vi "SettingsPanel.vi"(8 "error in":errorcluster, 11 "Settings In":T2={"Harware Configuration"={"Camera"="cam1", "Frames Per Second"=15, "Simulate Recording"=FALSE, "Simulated Recording Sample"=path "", "Timestamp Method"=enum."Camera Timestamp"}, "Base Recording Path"=path "", "Type Of Recording"="", "Recording Codec"="", "TrackingSettings"={"Max Radius"=10, "Threshold"=160.0, "ROI"={"Left"=0, "Top"=0, "Right"=0, "Bottom"=0, "Rotation"=0.0}}, "Calibration"={"Pixel Width (X)"=1.0, "Pixel Height (Y)"=1.0}, "Broadcast Length"=0} {"Broadcast Length" min=0; "TrackingSettings"."ROI"."Rotation" format="%.2f"; "TrackingSettings"."ROI"."Left" scale=0.0..1024.0; "TrackingSettings"."ROI"."Right" scale=0.0..1024.0; "TrackingSettings"."Threshold" scale=0.0..255.0}) -> (0 "error out":errorcluster, 2 "Canceled?":bool, 3 "Settings Out":T2={"Harware Configuration"={"Camera"="cam1", "Frames Per Second"=15, "Simulate Recording"=FALSE, "Simulated Recording Sample"=path "", "Timestamp Method"=enum."Camera Timestamp"}, "Base Recording Path"=path "", "Type Of Recording"="", "Recording Codec"="", "TrackingSettings"={"Max Radius"=0, "Threshold"=160.0, "ROI"={"Left"=0, "Top"=0, "Right"=0, "Bottom"=0, "Rotation"=0.0}}, "Calibration"={"Pixel Width (X)"=1.0, "Pixel Height (Y)"=1.0}, "Broadcast Length"=0} {"Broadcast Length" min=0; "TrackingSettings"."ROI"."Rotation" format="%.2f"; "TrackingSettings"."ROI"."Left" scale=0.0..1024.0; "TrackingSettings"."ROI"."Right" scale=0.0..1024.0; "TrackingSettings"."Threshold" scale=0.0..255.0})   [LabVIEW 2017, in "ImageAcquisitionLibrary.lvlib"]
uses:
  ImageAcquisitionLibrary.lvlib
  <vilib>/userdefined/High Color/IMAQdx.ctl
  Settings.ctl
  Tracking/TrackingSettings.ctl
  Calibration.ctl
panel:
  in  "Calibration":T1={"Pixel Width (X)"=1.0, "Pixel Height (Y)"=1.0} {"Pixel Width (X)" format="%.0p"; "Pixel Height (Y)" format="%.0p"}
  in  "Tracking Settings":bool
  in  "Type Of Recording":string(combo)="Snapshot"
  in  "fps":dbl=15.0
  in  "Camera":T3
  in  "Simulate":bool
  in  "Simulated Acquisition Sample":path=path "D:/Dropbox/Colloids/2015-06-15/ImageAcquisitionProgram/SimulationInput/SampleImage.jpg"
  in  "Recording Path":path=path "C:/Users/aortiza/Desktop"
  in  "Codex":string(combo)="Y800 Uncompressed Grey Scale (NI Vision)"
  in  "Cancel Button":bool
  in  "OK Button":bool
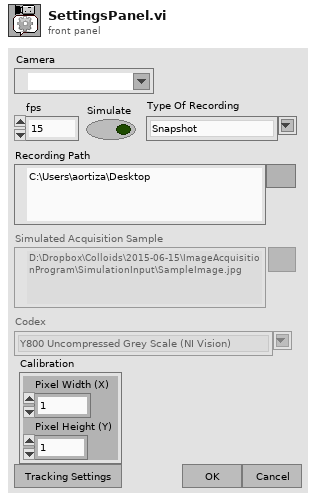
[diagram p1: front panel]
types:
  T1 = typedef "ImageAcquisitionLibrary.lvlib/Calibration.ctl" = cluster{"Pixel Width (X)":dbl, "Pixel Height (Y)":dbl}
  T2 = typedef "ImageAcquisitionLibrary.lvlib/Settings.ctl" = cluster{"Harware Configuration":cluster{"Camera":T3, "Frames Per Second":u32, "Simulate Recording":bool, "Simulated Recording Sample":path, "Timestamp Method":enum16{"System Timestamp", "Camera Timestamp", "IMAQdx Timestamp"}}, "Base Recording Path":path, "Type Of Recording":string, "Recording Codec":string, "TrackingSettings":T4, "Calibration":T1, "Broadcast Length":i32}
  T3 = typedef "IMAQdx.ctl" = refnum<k21>
  T4 = typedef "ImageAcquisitionLibrary.lvlib/TrackingSettings.ctl" = cluster{"Max Radius":i32, "Threshold":sgl, "ROI":T5}
  T5 = typedef "IMAQ Rectangle" = cluster{"Left":i32, "Top":i32, "Right":i32, "Bottom":i32, "Rotation":dbl}
  T6 = typedef "Image Type" = u32
  T7 = typedef "IMAQ Image.ctl" = refnum<image>
  T8 = enum8{"Enabled", "Disabled", "Disabled and Grayed Out"}
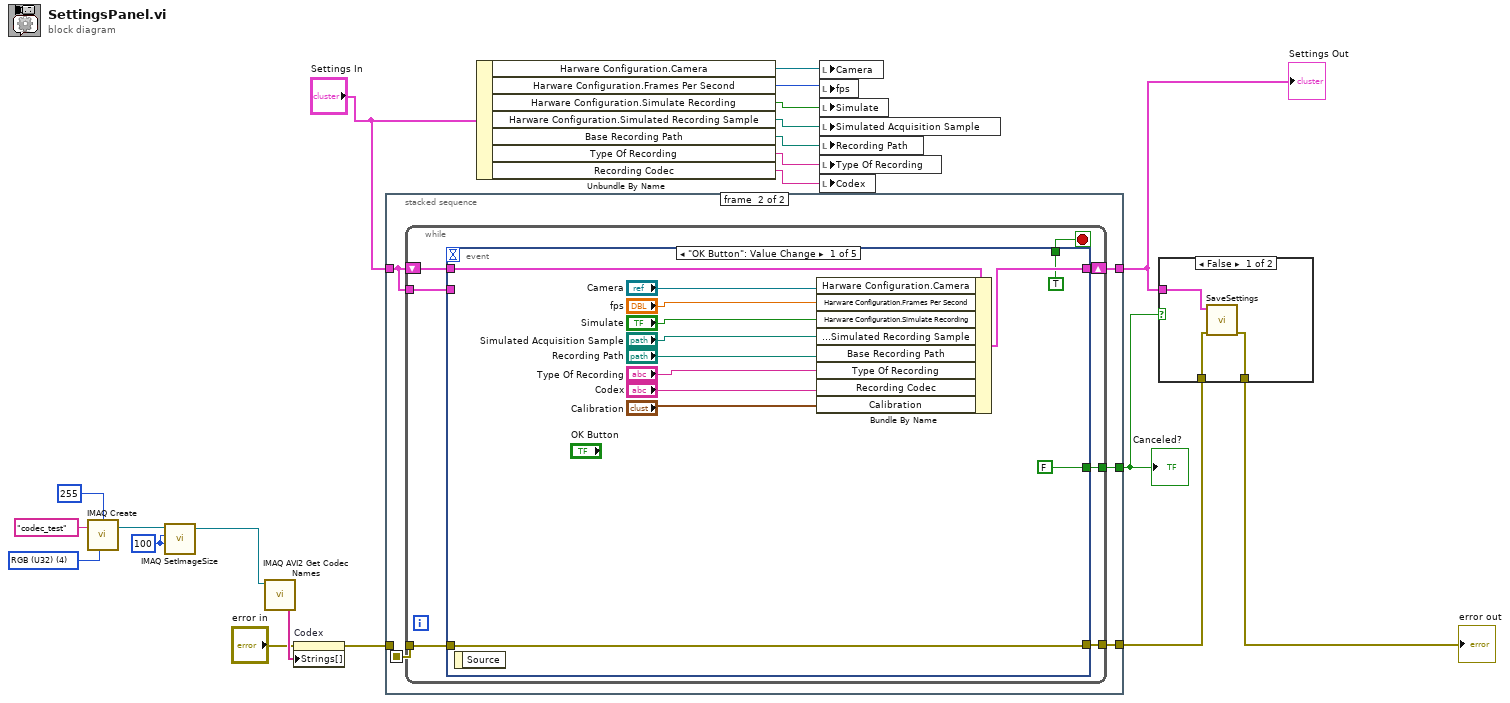
[diagram p0: block diagram]
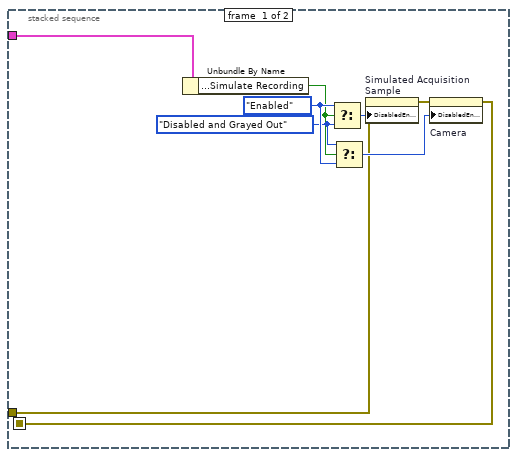
[diagram p2: hidden frame]
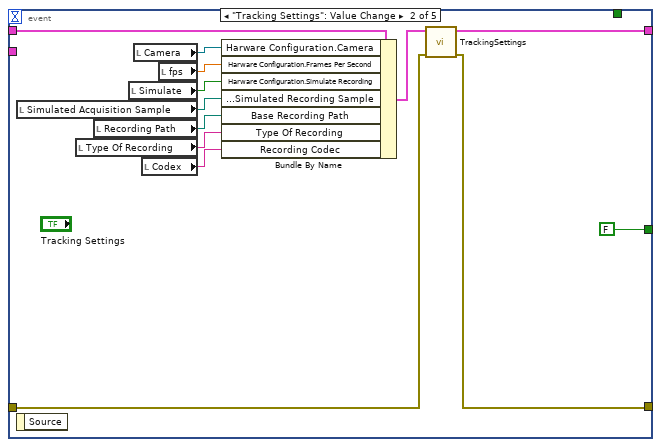
[diagram p3: hidden frame]
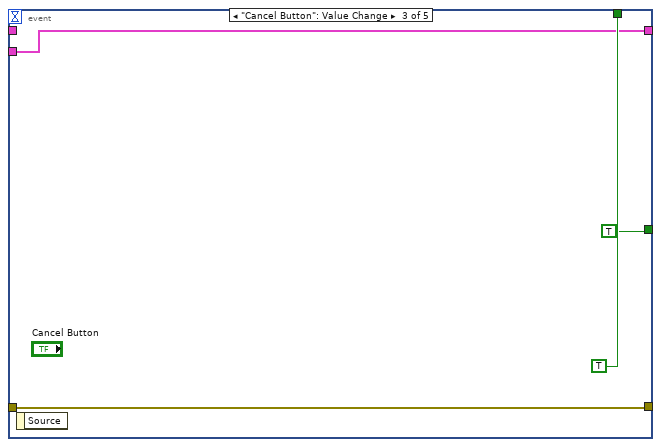
[diagram p4: hidden frame]
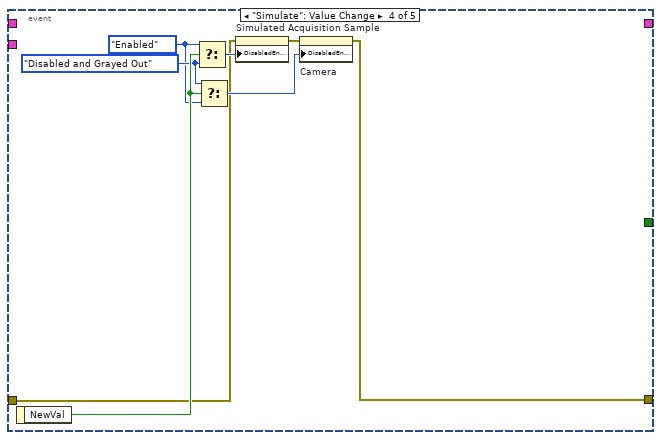
[diagram p5: hidden frame]
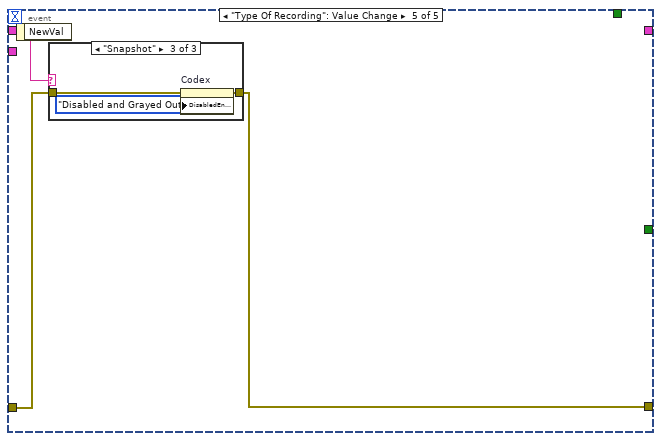
[diagram p6: hidden frame]
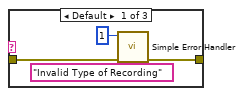
[diagram p7: hidden frame]
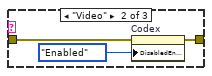
[diagram p8: hidden frame]
diagram:
  w3 = 100 ("X Resolution")
  w6 = T6 4 items=["Grayscale (U8)", "Grayscale (I16)", "Grayscale (SGL)", "Complex (CSG)", "RGB (U32)", "HSL (U32)", "RGB (U64)", "Grayscale (U16)"] ("Image Type")
  n1 = call "IMAQ Create"("Border Size"=255, "Image Name"="codec_test", "Image Type"=w6) -> ("New Image"=w2:T7)  [unwired: 2 in, 1 out]
  n2 = call "IMAQ SetImageSize"("Y Resolution"=w3, "X Resolution"=w3, "Image"=w2) -> ("Image Out"=w1:T7)  [unwired: 2 in, 1 out]
  n3 = call "IMAQ AVI2 Get Codec Names"("Image"=w1) -> ("Codec Names"=w13:string[])  [unwired: 9 in, 1 out]
  n4 = property on="Codex" class="CmbBox"(error in="error in", "Strings[]"=w13) -> (error out=w11:errorcluster)  [unwired: 1 in, 1 out]
  n5 = stacked-sequence {
    seq-local: [w22 _] -> [_ w32]
    tunnel: "Settings In" -> [w26 w31]
    tunnel: w11 -> [w23 _]
    tunnel: [_ w35] -> w7
    tunnel: [_ w34] -> w10
    tunnel: [_ w33] -> w9
    frame #0 {
      w24 = T8."Disabled and Grayed Out" ("Disabled")
      w27 = T8."Enabled" ("Disabled")
      n6 = Unbundle By Name(w26) -> ("Harware Configuration.Simulate Recording"=w25:bool)
      n7 = Select(t=w27, s=w25, f=w24) -> (s? t:f=w30:T8)
      n8 = Select(t=w24, s=w25, f=w27) -> (s? t:f=w29:T8)
      n9 = property on="Simulated Acquisition Sample" class="Path"(error in=w23, "DisabledEnum"=w30) -> (error out=w28:errorcluster)  [unwired: 1 in, 1 out]
      n10 = property on="Camera" class="IMAQdx (strict)"(error in=w28, "DisabledEnum"=w29) -> (error out=w22:errorcluster)  [unwired: 1 in, 1 out]
    }
    frame #1 {
      n11 = while {
        shift-right: [w36] -> w34
        shift-left: w31 -> [w42]
        tunnel: [w40] -> w35
        tunnel: [w39] -> w33
        tunnel: w32 -> [w38]
        tunnel: w31 -> [w37]
        stop <- w41 stop-if-true
        n12 = event shown="[0] \"OK Button\": Value Change" {
          selector: _ -> [_ _ _ _ _]
          dyn-events: _ -> [_ _ _ _ _]
          timeout: _ -> [_ _ _ _ _]
          tunnel: w42 -> [w55 w68 _ _ _]
          tunnel: [TRUE _ TRUE _ _] -> w41
          tunnel: [FALSE FALSE TRUE _ _] -> w40
          tunnel: [w43 w63 w70 w76 w82] -> w39
          tunnel: w38 -> [w43 w64 w70 w73 w81]
          tunnel: w37 -> [_ _ w69 _ _]
          tunnel: [w50 w65 w69 _ _] -> w36
          event "OK Button": Value Change {
            n13 = event-data() -> ()  [unwired: 1 in, 1 out]
            n14 = Bundle By Name(cluster=w55, "Harware Configuration.Camera"="Camera", "Harware Configuration.Frames Per Second"="fps", "Harware Configuration.Simulate Recording"="Simulate", "Harware Configuration.Simulated Recording Sample"="Simulated Acquisition Sample", "Base Recording Path"="Recording Path", "Type Of Recording"="Type Of Recording", "Recording Codec"="Codex", "Calibration"="Calibration") -> (w50:T2)
          }
          event "Tracking Settings": Value Change {
            n15 = local read "Simulated Acquisition Sample"() -> (w59:path)
            n16 = event-data() -> ()  [unwired: 1 in, 1 out]
            n17 = local read "Type Of Recording"() -> (w61:string)
            n18 = local read "Recording Path"() -> (w60:path)
            n19 = local read "Simulate"() -> (w58:bool)
            n20 = local read "Camera"() -> (w56:T3)
            n21 = local read "Codex"() -> (w62:string)
            n22 = local read "fps"() -> (w57:dbl)
            n23 = Bundle By Name(cluster=w68, "Harware Configuration.Camera"=w56, "Harware Configuration.Frames Per Second"=w57, "Harware Configuration.Simulate Recording"=w58, "Harware Configuration.Simulated Recording Sample"=w59, "Base Recording Path"=w60, "Type Of Recording"=w61, "Recording Codec"=w62) -> (w66:T2)
            n24 = call "TrackingSettings.vi"("error in"=w64, "Settings In"=w66) -> ("error out"=w63:errorcluster, "Settings Out"=w65:T2)  [unwired: 7 in, 1 out]
          }
          event "Cancel Button": Value Change {
            n25 = event-data() -> ()  [unwired: 1 in, 1 out]
          }
          event "Simulate": Value Change {
            w75 = T8."Disabled and Grayed Out" ("Disabled")
            w74 = T8."Enabled" ("Disabled")
            n26 = event-data() -> ("NewVal"=w79:bool)  [unwired: 1 in]
            n27 = Select(t=w74, s=w79, f=w75) -> (s? t:f=w80:T8)
            n28 = Select(t=w75, s=w79, f=w74) -> (s? t:f=w78:T8)
            n29 = property on="Simulated Acquisition Sample" class="Path"(error in=w73, "DisabledEnum"=w80) -> (error out=w77:errorcluster)  [unwired: 1 in, 1 out]
            n30 = property on="Camera" class="IMAQdx (strict)"(error in=w77, "DisabledEnum"=w78) -> (error out=w76:errorcluster)  [unwired: 1 in, 1 out]
          }
          event "Type Of Recording": Value Change {
            n31 = event-data() -> ("NewVal"=w83:string)  [unwired: 1 in]
            n32 = case shown="\"Snapshot\"" w83 {
              tunnel: [w86 w88 w92] -> w82
              tunnel: w81 -> [w87 w89 w91]
              frame Default {
                n33 = call <vilib>:"Simple Error Handler.vi"("error code (no error:0)"=1, "error source (\" \")"="Invalid Type of Recording" ("error source (\" \")"), "error in (no error)"=w87) -> ("error out"=w86:errorcluster)  [unwired: 2 in, 4 out]
              }
              frame "Video" {
                n34 = property on="Codex" class="CmbBox"(error in=w89, "DisabledEnum"=T8."Enabled" ("Disabled")) -> (error out=w88:errorcluster)  [unwired: 1 in, 1 out]
              }
              frame "Snapshot" {
                n35 = property on="Codex" class="CmbBox"(error in=w91, "DisabledEnum"=T8."Disabled and Grayed Out" ("Disabled")) -> (error out=w92:errorcluster)  [unwired: 1 in, 1 out]
              }
            }
          }
        }
      }
    }
  }
  "Settings Out" <- w10
  "Canceled?" <- w7
  n36 = Unbundle By Name("Settings In") -> ("Harware Configuration.Camera"=w20:T3, "Harware Configuration.Frames Per Second"=w19:u32, "Harware Configuration.Simulate Recording"=w18:bool, "Harware Configuration.Simulated Recording Sample"=w16:path, "Base Recording Path"=w17:path, "Type Of Recording"=w15:string, "Recording Codec"=w14:string)
  n37 = local write "Camera"(w20) -> ()
  n38 = local write "fps"(w19) -> ()
  n39 = local write "Simulate"(w18) -> ()
  n40 = local write "Simulated Acquisition Sample"(w16) -> ()
  n41 = local write "Recording Path"(w17) -> ()
  n42 = local write "Type Of Recording"(w15) -> ()
  n43 = local write "Codex"(w14) -> ()
  n44 = case shown="False" w7 {
    tunnel: w10 -> [w96 _]
    tunnel: w9 -> [w95 w97]
    tunnel: [w94 w97] -> w8
    frame False {
      n45 = call "SaveSettings.vi"("error in (no error)"=w95, "Settings"=w96) -> ("error out"=w94:errorcluster)  [unwired: 9 in]
    }
    frame True {
    }
  }
  "error out" <- w8
